vi "Write purgeFlow.vi"(8 "error in (no error)":errorcluster, 10 "Alicat Device":refnum<class "Alicat Device.lvclass">, 11 "tCRD in":refnum<class "Aircraft OPCCRD.lvclass">) -> (0 "error out":errorcluster, 3 "tCRD out":refnum<class "Aircraft OPCCRD.lvclass">)   [LabVIEW 2015, in "Aircraft OPCCRD.lvclass"]
uses:
  Aircraft OPCCRD.lvclass
  Devices/Alicat/Session Based/Alicat Device.lvclass
  Aircraft OPCCRD.lvclass/Aircraft OPCCRD.ctl
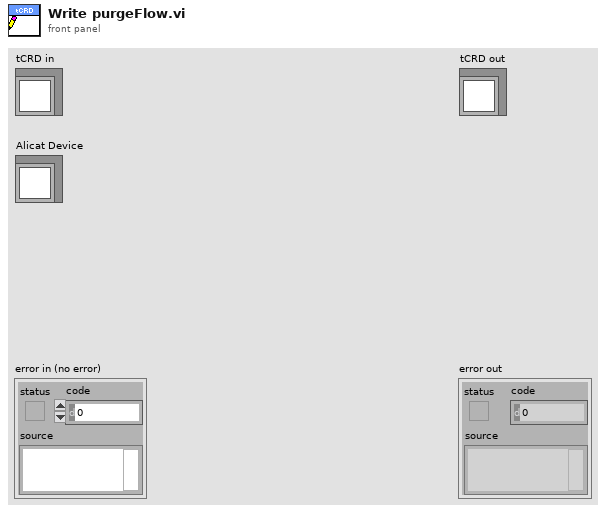
[diagram p1: front panel]
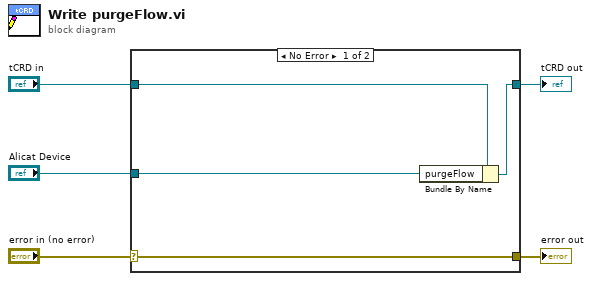
[diagram p0: block diagram]
diagram:
  n1 = case shown="No Error" "error in (no error)" {
    selector: "error in (no error)" -> [w9 w10]
    tunnel: [w9 w10] -> w4
    tunnel: [w7 w11] -> w2
    tunnel: "tCRD in" -> [w8 w11]
    tunnel: "Alicat Device" -> [w6 _]
    frame No Error {
      n2 = Bundle By Name(cluster=w8, "purgeFlow"=w6) -> (w7:refnum<class "Aircraft OPCCRD.lvclass">)
    }
    frame Error {
    }
  }
  "error out" <- w4
  "tCRD out" <- w2
